vi "cm_Set Channel Names.vi"(0 "Display State In":T1={"Chan"=[], "First Drop?"=FALSE, "Notifier Name"="", "Refresh View"=FALSE, "Scale to Input Range"=FALSE, "Linear View"=FALSE, "Display"={"Current"=6618880, "Peak"=6618880}, "Property/Method"=enum."No Update", "Time Display Ref"=[]}, 5 "Channel Index":i32[](array[numeric]), 7 "Channel Name":string[](array[string]), 9 "Container State":T3, 11 "error in (no error)":errorcluster) -> (4 "Display State Out":T1={"Chan"=[], "First Drop?"=FALSE, "Notifier Name"="", "Refresh View"=FALSE, "Scale to Input Range"=FALSE, "Linear View"=FALSE, "Display"={"Current"=6618880, "Peak"=6618880}, "Property/Method"=enum."No Update", "Time Display Ref"=[]}, 15 "error out":errorcluster)   [LabVIEW 2012, in "Channel Monitor.xctl"]
doc: "Set the channel name for one or more channels of the Channel Monitor XControl. The default channel name is the Channel Name attribute found in the waveform datatype."
uses:
  Channel Monitor.xctl
  <vilib>/_xctls/Container State.ctl
  subVIs/cm_Channel Monitor State.ctl
  TypeDef/cm_Property_Method.ctl
  <vilib>/_xctls/XControlSupport.lvlib
panel:
  # "Add Controls & Indicators that form the parameters of the method here. Hook them to the connector pane. Do not delete the controls & indicators that are already hooked to the connector pane.\n \nTo setup the parameters  for this method, right click on this item in the Project Tree & select \"Configure Method...\"."
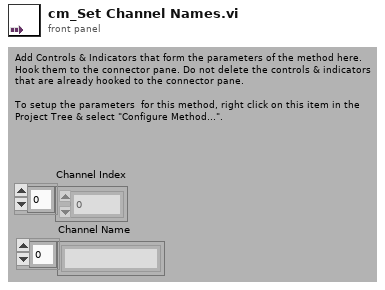
[diagram p1: front panel]
types:
  T1 = typedef "Channel Monitor.xctl/cm_Channel Monitor State.ctl" = cluster{"Chan":cluster{"ChanName":string, "Current":dbl, "Peak":dbl, "Input Range":dbl}[], "First Drop?":bool, "Notifier Name":string, "Refresh View":bool, "Scale to Input Range":bool, "Linear View":bool, "Display":cluster{"Current":u32, "Peak":u32}, "Property/Method":T2, "Time Display Ref":refnum<vi>[]}
  T2 = typedef "Channel Monitor.xctl/cm_Property_Method.ctl" = enum16{"No Update", "Color: Currrent", "Color: Peak", "Close Time Displays"}
  T3 = typedef "XControlSupport.lvlib/Container State.ctl" = cluster{"Indicator?":bool, "Run Mode?":bool, " Refnum":refnum<vi>}
  T4 = cluster{"ChanName":string, "Current":dbl, "Peak":dbl, "Input Range":dbl}[]
  T5 = cluster{"ChanName":string, "Current":dbl, "Peak":dbl, "Input Range":dbl}
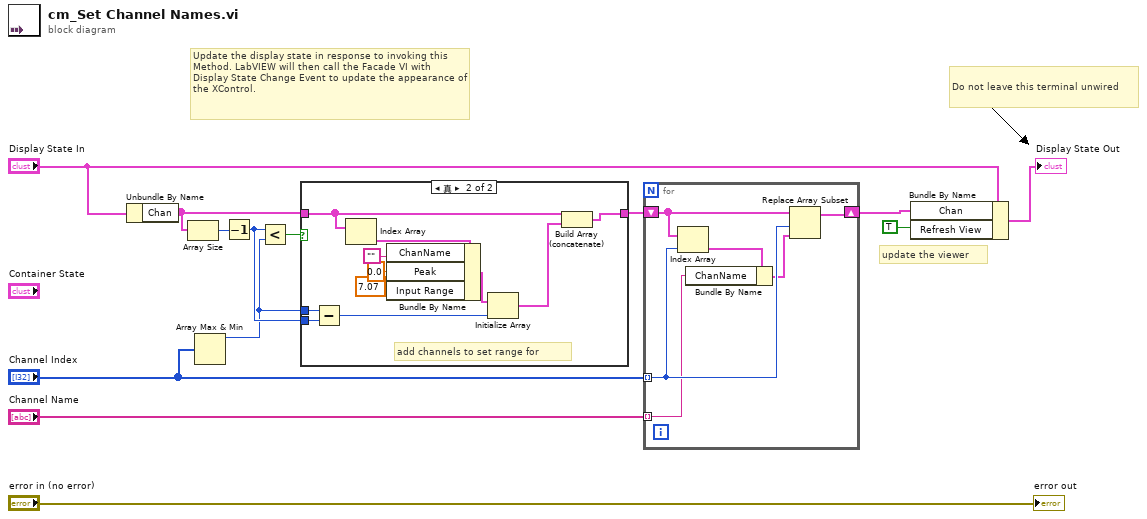
[diagram p0: block diagram]
diagram:
  # "update the viewer"
  # "Do not leave this terminal unwired"
  # "Update the display state in response to invoking this Method. LabVIEW will then call the Facade VI with Display State Change Event to update the appearance of the XControl."
  n1 = Unbundle By Name("Display State In") -> ("Chan"=w11:T4)
  n2 = Array Size(array=w11) -> (size(s)=w12:i32)
  n3 = Array Max & Min(array="Channel Index") -> (max value=w8:i32)  [unwired: 3 out]
  n4 = Decrement(x=w12) -> (x-1=w9:i32)
  n5 = Less?(x=w9, y=w8) -> (x < y?=w10:bool)
  n6 = case shown="真" w10 {
    tunnel: w11 -> [w14 w17]
    tunnel: w9 -> [_ w25]
    tunnel: w8 -> [_ w24]
    tunnel: [w14 w16] -> w7
    frame False {
    }
    frame True {
      # "add channels to set range for"
      n7 = Subtract(x=w24, y=w25) -> (x-y=w18:i32)
      n8 = Index Array(array=w17) -> (element=w23:T5)  [unwired: 1 in]
      n9 = Bundle By Name(cluster=w23, "ChanName"="", "Peak"=0.0, "Input Range"=7.07) -> (w19:T5)
      n10 = Initialize Array(w19, w18) -> (w15:T4)
      n11 = Build Array (concatenate)(w17, w15) -> (w16:T4)
    }
  }
  n12 = for {
    tunnel: "Channel Index" -> [w28] mode=indexing
    shift-right: [w31] -> w6
    shift-left: w7 -> [w30]
    tunnel: "Channel Name" -> [w26] mode=indexing
    n13 = Index Array(array=w30, index=w28) -> (element=w29:T5)
    n14 = Bundle By Name(cluster=w29, "ChanName"=w26) -> (w27:T5)
    n15 = Replace Array Subset(array=w30, new element=w27, index=w28) -> (w31:T4)
  }
  n16 = Bundle By Name(cluster="Display State In", "Chan"=w6, "Refresh View"=TRUE) -> (→"Display State Out":T1)
  "error out" <- "error in (no error)"
